vi "is a.vi"(8 "error in (no error)":errorcluster, 11 "PXI 4070 in":refnum<class "PXI 4070.lvclass">) -> (0 "error out":errorcluster, 2 "is a":string, 3 "PXI 4070 out":refnum<class "PXI 4070.lvclass">)   [LabVIEW 2013, in "PXI 4070.lvclass"]
uses:
  PXI 4070.lvclass
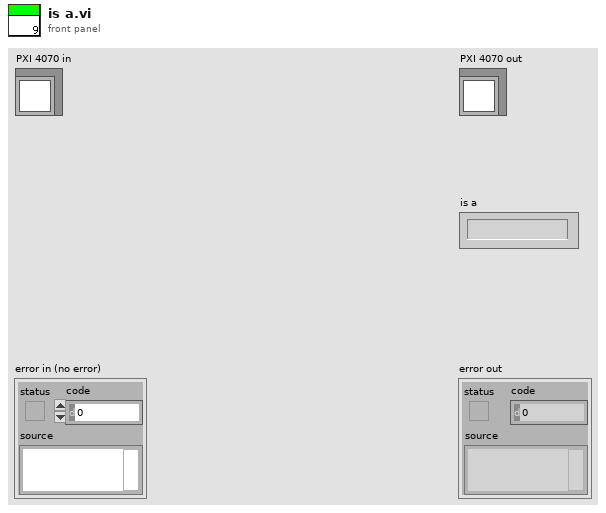
[diagram p1: front panel]
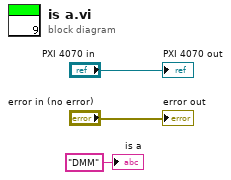
[diagram p0: block diagram]
diagram:
  "error out" <- "error in (no error)"
  "PXI 4070 out" <- "PXI 4070 in"
  "is a" <- "DMM" ("is a")
